vi "database_connection_test.vi"() -> ()   [LabVIEW 2015]
panel:
  out "error out":errorcluster
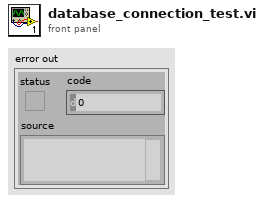
[diagram p1: front panel]
types:
  T1 = typedef "NI_Database_API.lvlib/Conn ObjectReference.ctl" = refnum<k1>
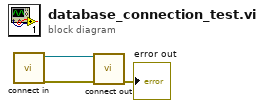
[diagram p0: block diagram]
diagram:
  n1 = call "connect in.vi"() -> ("error out"=w2:errorcluster, "Database Connection"=w3:T1)  [unwired: 7 in, 1 out]
  n2 = call "connect out.vi"("error in (no error)"=w2, "connection reference"=w3) -> ("error out"=→"error out":errorcluster)  [unwired: 9 in]
